vi "Auto State Machine.vi"   [LabVIEW 2013]
uses:
  typedefs/singleUseSubstate.ctl
  typedefs/subStates.ctl
  typedefs/DevRef Type.ctl
  typedefs/fg_typedef.ctl
  <vilib>/Rock Robotics/WPI/Solenoid/WPI_SolenoidValue.ctl
  <vilib>/Rock Robotics/WPI/Solenoid/WPI_SolenoidGetEnum.vi
panel:
  # "A State Machine to Handle One or Two Ball Autonomous"
types:
  T1 = typedef "singleUseSubstate.ctl" = enum16{"null", "wait", "shift high", "shift low", "extend shooter", "retract shooter", "latch", "unlatch"}
  T2 = typedef "subStates.ctl" = enum16{"null", "wait", "driver control", "auto", "manual override", "hold position", "rotate", "pickup", "pass", "load", "goto shoot", "shoot high goal", "shoot low goal", "cancel arm", "cancel shooter", "end"}
  T3 = typedef "WPI_SolenoidValue.ctl" = enum16{"Off", "On", "Forward", "Reverse"}
  T4 = typedef "DevRef Type.ctl" = enum16{"Shooter Solenoid", "Latch Solenoid", "Right Up Sensor", "Right Down Sensor", "Hold Sensor", "Arm Encoder"}
  T5 = typedef "fg_typedef.ctl" = enum16{"Get", "Set"}
  T6 = typedef "WPI_DigitalInputDevRef.ctl" = cluster{"DevStatus":errorcluster, "DIO Channel":T7, "Digital Module":T8}
  T7 = typedef "FPGA_DIOChannel.ctl" = enum8{"DIO 1", "DIO 2", "DIO 3", "DIO 4", "DIO 5", "DIO 6", "DIO 7", "DIO 8", "DIO 9", "DIO 10", "DIO 11", "DIO 12", "DIO 13", "DIO 14", "Invalid"}
  T8 = typedef "FPGA_TypedefDigitalModule.ctl" = enum16{"Digital Module 1", "Digital Module 2"}
  T9 = typedef "WPI_SolenoidDevRef.ctl" = cluster{"DevStatus":errorcluster, "Solenoid Module":T10, "Forward Solenoid Channel":T11, "Reverse Solenoid Channel":T11}
  T10 = typedef "FPGA_TypedefSolenoidModule.ctl" = enum16{"Solenoid Module 1", "Solenoid Module 2"}
  T11 = typedef "WPI_SolenoidChannel.ctl" = enum8{"Solenoid 1", "Solenoid 2", "Solenoid 3", "Solenoid 4", "Solenoid 5", "Solenoid 6", "Solenoid 7", "Solenoid 8", "Invalid"}
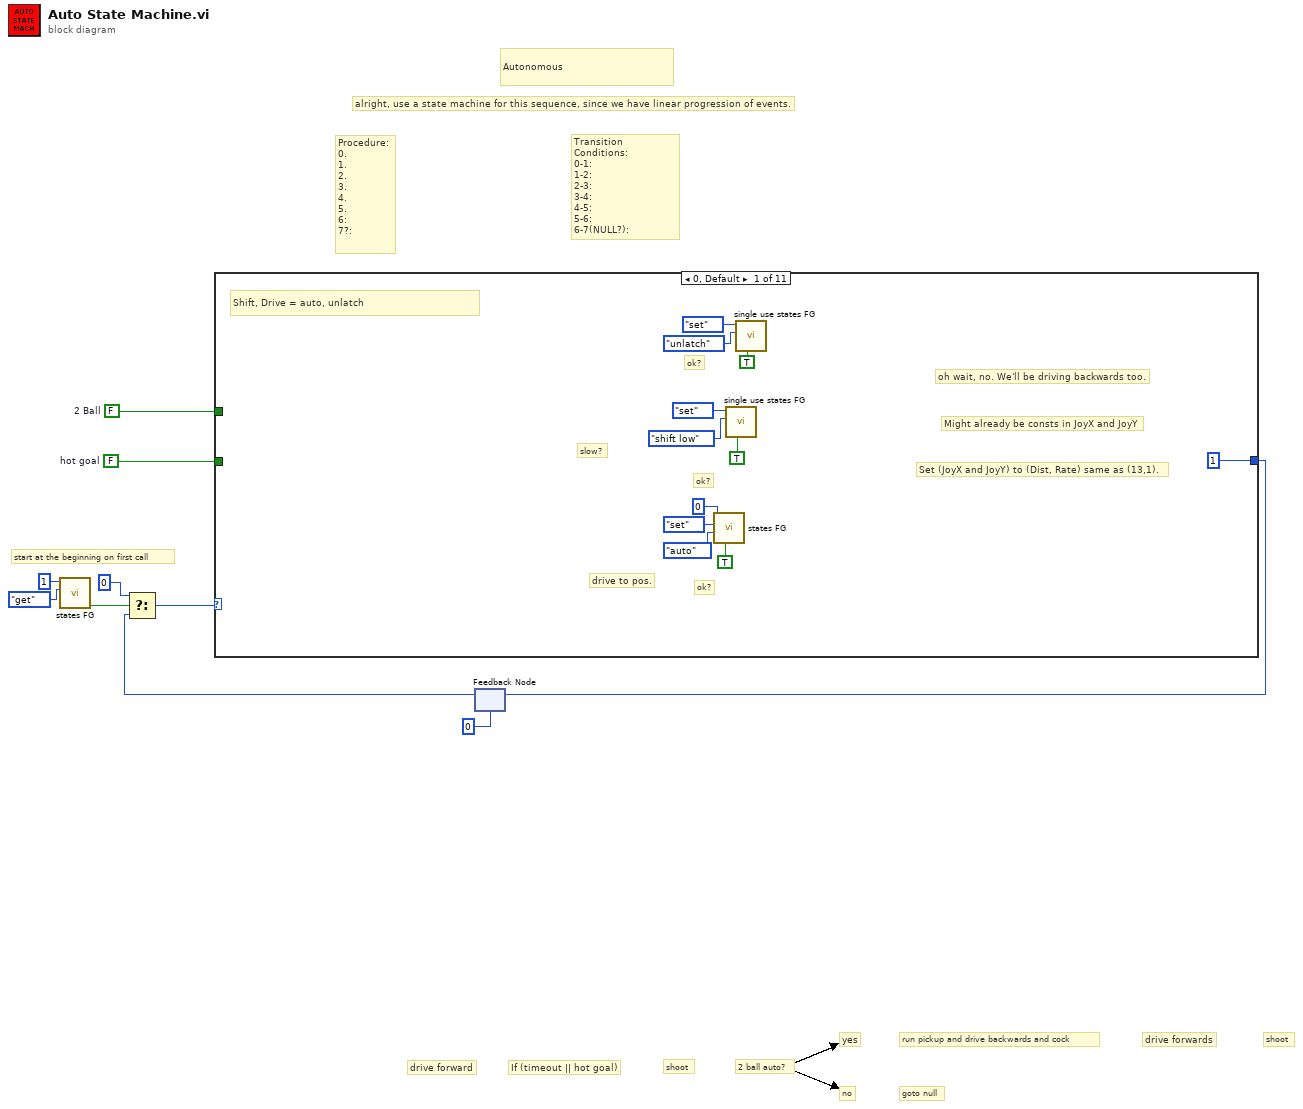
[diagram p0: block diagram]
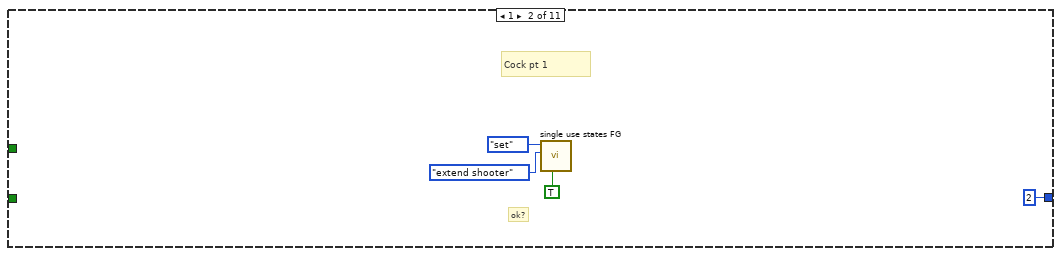
[diagram p2: hidden frame]
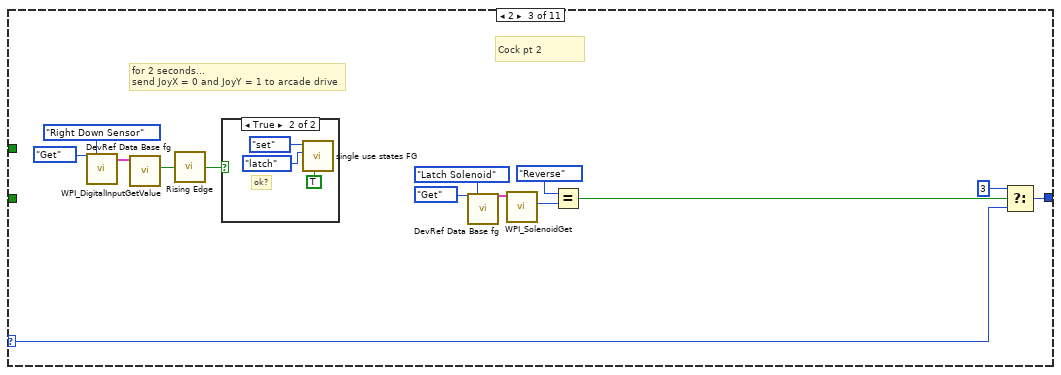
[diagram p3: hidden frame]
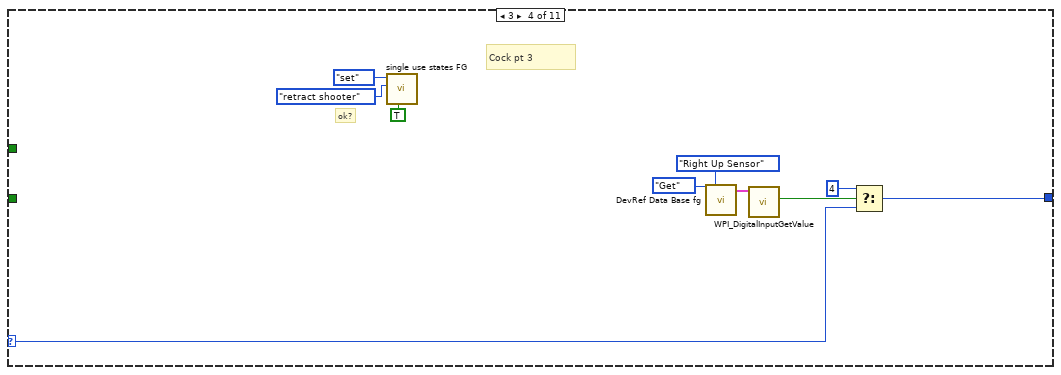
[diagram p5: hidden frame]
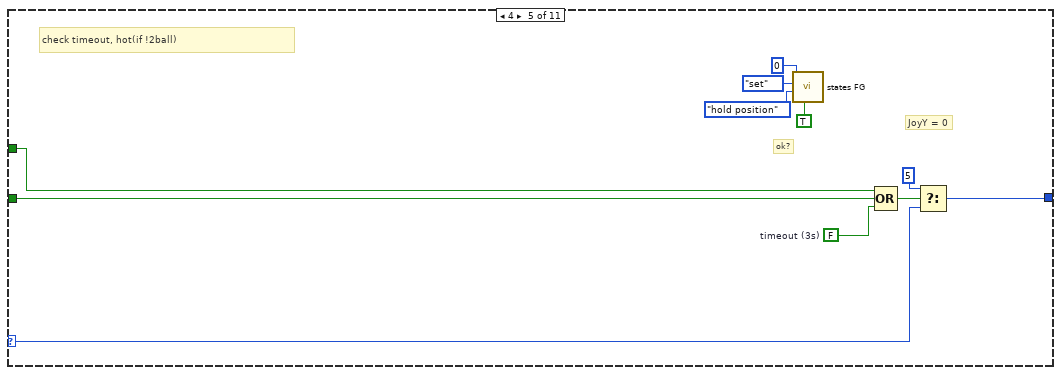
[diagram p6: hidden frame]
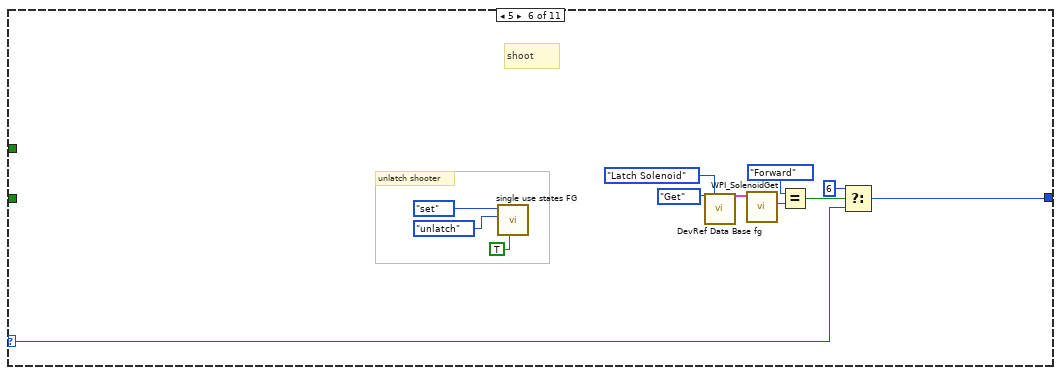
[diagram p7: hidden frame]
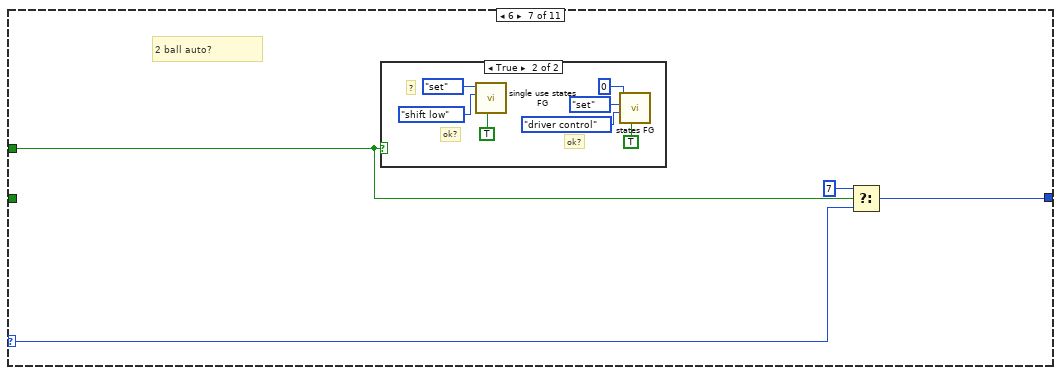
[diagram p8: hidden frame]
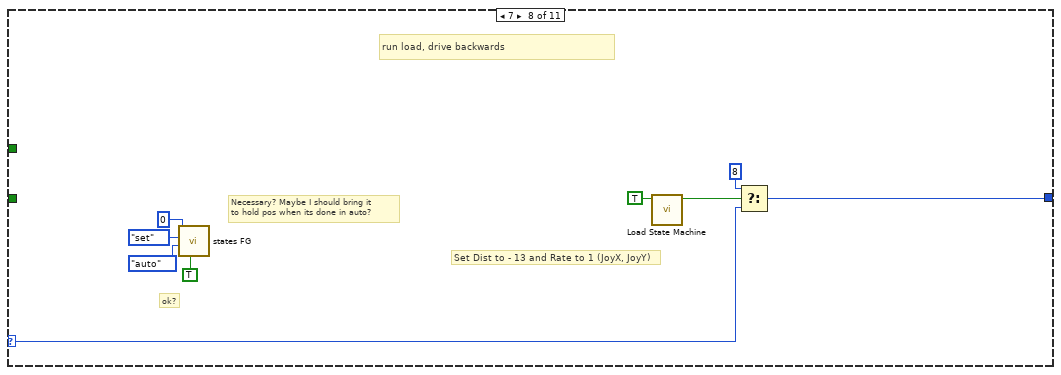
[diagram p10: hidden frame]
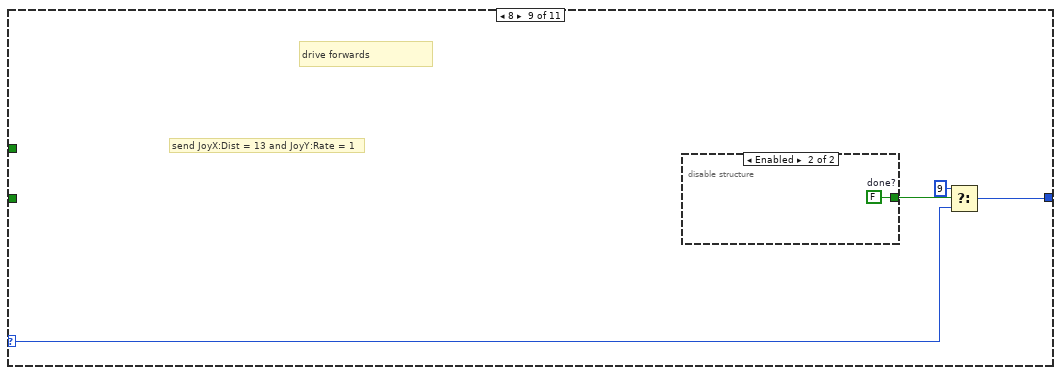
[diagram p11: hidden frame]
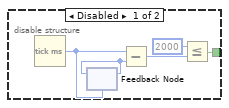
[diagram p12: hidden frame]
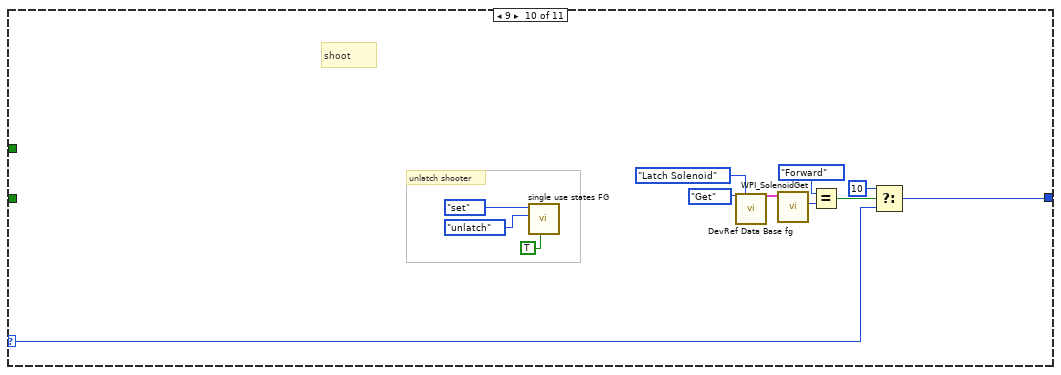
[diagram p13: hidden frame]
diagram:
  w3 = FALSE  # hot goal
  w4 = FALSE  # 2 Ball
  # "2 ball auto?"
  # "goto null"
  # "shoot"
  # "drive forwards"
  # "run pickup and drive backwards and cock"
  # "If (timeout || hot goal)"
  # "shoot"
  # "drive forward"
  # "no"
  # "yes"
  # "Transition Conditions:\n0-1: \n1-2: \n2-3: \n3-4: \n4-5: \n5-6:\n6-7(NULL?):"
  # "start at the beginning on first call"
  # "Autonomous"
  # "Procedure: \n0. \n1.\n2. \n3. \n4. \n5.\n6:\n7?:"
  # "alright, use a state machine for this sequence, since we have linear progression of events."
  n1 = call "states FG.vi"("menu (get)"=enum16{"set", "get"}."get", "Loop ID"=1) -> ("first call?"=w5:bool)  [unwired: 6 in, 3 out]
  n2 = feedback #1(u8 0) -> (w6:u8)
  n3 = Select(t=u8 0, s=w5, f=w6) -> (s? t:f=w8:u8)
  n4 = case shown="0, Default" w8 {
    selector: w8 -> [_ _ w39 w46 w63 w66 w79 w95 w97 w107 w118]
    tunnel: w4 -> [_ _ _ _ w59 _ w76 _ _ _ _]
    tunnel: w3 -> [_ _ _ _ w58 _ _ _ _ _ _]
    tunnel: [u8 1 u8 2 ("t") w38 w45 w57 w64 w77 w92 w96 w106 w118] -> w1
    frame 0, Default {
      # "oh wait, no. We'll be driving backwards too."
      # "Might already be consts in JoyX and JoyY"
      # "drive to pos."
      # "ok?"
      # "Shift, Drive = auto, unlatch"
      # "Set (JoyX and JoyY) to (Dist, Rate) same as (13,1)."
      # "ok?"
      # "ok?"
      # "slow?"
      n5 = call "states FG.vi"("exit in"=TRUE, "subState in"=subStates."auto", "menu (get)"=enum16{"set", "get"}."set", "Loop ID"=0) -> ()  [unwired: 4 in, 4 out]
      n6 = call "single use states FG.vi"("exit in"=TRUE, "substate"=singleUseSubstate."shift low", "menu (get)"=enum16{"set", "get"}."set") -> ()  [unwired: 5 in, 4 out]
      n7 = call "single use states FG.vi"("exit in"=TRUE, "substate"=singleUseSubstate."unlatch", "menu (get)"=enum16{"set", "get"}."set") -> ()  [unwired: 5 in, 4 out]
    }
    frame 1 {
      # "Cock pt 1"
      # "ok?"
      n8 = call "single use states FG.vi"("exit in"=TRUE, "substate"=singleUseSubstate."extend shooter", "menu (get)"=enum16{"set", "get"}."set") -> ()  [unwired: 5 in, 4 out]
    }
    frame 2 {
      # "for 2 seconds...\nsend JoyX = 0 and JoyY = 1 to arcade drive"
      # "Cock pt 2"
      n9 = call "DevRef Data Base fg.vi"("Menu"=fg_typedef."Get", "DevRef to Get"=DevRef_Type."Right Down Sensor") -> ("Selected Sensor"=w35:T6)  [unwired: 23 in, 2 out]
      n10 = call <vilib>:"WPI_DigitalInputGetValue.vi"("DigitalInputDevRef"=w35) -> ("Value"=w33:bool)  [unwired: 8 in, 2 out]
      n11 = call "Rising Edge.vi"("Input"=w33) -> ("Rising Edge"=w34:bool)
      n12 = case shown="True" w34 {
        frame False {
        }
        frame True {
          # "ok?"
          n13 = call "single use states FG.vi"("exit in"=TRUE, "substate"=singleUseSubstate."latch", "menu (get)"=enum16{"set", "get"}."set") -> ()  [unwired: 5 in, 4 out]
        }
      }
      n14 = call "DevRef Data Base fg.vi"("Menu"=fg_typedef."Get", "DevRef to Get"=DevRef_Type."Latch Solenoid") -> ("Selected Solenoid"=w30:T9)  [unwired: 23 in, 2 out]
      n15 = call-poly <vilib>:"WPI_SolenoidGet.vi"("SolenoidDevRef"=w30) -> ("Value"=w29:T3)  [unwired: 8 in, 2 out]
      n16 = Equal?(x=WPI_SolenoidValue."Reverse", y=w29) -> (x = y?=w26:bool)
      n17 = Select(t=u8 3, s=w26, f=w39) -> (s? t:f=w38:u8)
    }
    frame 3 {
      # "Cock pt 3"
      # "ok?"
      n18 = call "single use states FG.vi"("exit in"=TRUE, "substate"=singleUseSubstate."retract shooter", "menu (get)"=enum16{"set", "get"}."set") -> ()  [unwired: 5 in, 4 out]
      n19 = call "DevRef Data Base fg.vi"("Menu"=fg_typedef."Get", "DevRef to Get"=DevRef_Type."Right Up Sensor") -> ("Selected Sensor"=w47:T6)  [unwired: 23 in, 2 out]
      n20 = call <vilib>:"WPI_DigitalInputGetValue.vi"("DigitalInputDevRef"=w47) -> ("Value"=w44:bool)  [unwired: 8 in, 2 out]
      n21 = Select(t=u8 4, s=w44, f=w46) -> (s? t:f=w45:u8)
    }
    frame 4 {
      w60 = FALSE  # timeout (3s)
      # "ok?"
      # "JoyY = 0"
      # "check timeout, hot(if !2ball)"
      n22 = call "states FG.vi"("exit in"=TRUE, "subState in"=subStates."hold position", "menu (get)"=enum16{"set", "get"}."set", "Loop ID"=0) -> ()  [unwired: 4 in, 4 out]
      n23 = Compound Arithmetic op=OR(w59, w58, w60) -> (w61:bool)
      n24 = Select(t=u8 5, s=w61, f=w63) -> (s? t:f=w57:u8)
    }
    frame 5 {
      # "unlatch shooter"
      # "shoot"
      n25 = call "single use states FG.vi"("exit in"=TRUE, "substate"=singleUseSubstate."unlatch", "menu (get)"=enum16{"set", "get"}."set") -> ()  [unwired: 5 in, 4 out]
      n26 = call "DevRef Data Base fg.vi"("Menu"=fg_typedef."Get", "DevRef to Get"=DevRef_Type."Latch Solenoid") -> ("Selected Solenoid"=w71:T9)  [unwired: 23 in, 2 out]
      n27 = call-poly <vilib>:"WPI_SolenoidGet.vi"("SolenoidDevRef"=w71) -> ("Value"=w70:T3)  [unwired: 8 in, 2 out]
      n28 = Equal?(x=WPI_SolenoidValue."Forward" ("Value"), y=w70) -> (x = y?=w68:bool)
      n29 = Select(t=u8 6, s=w68, f=w66) -> (s? t:f=w64:u8)
    }
    frame 6 {
      # "2 ball auto?"
      n30 = case shown="True" w76 {
        frame False {
          # "goto null"
        }
        frame True {
          # "ok?"
          # "ok?"
          # "?"
          n31 = call "single use states FG.vi"("exit in"=TRUE, "substate"=singleUseSubstate."shift low", "menu (get)"=enum16{"set", "get"}."set") -> ()  [unwired: 5 in, 4 out]
          n32 = call "states FG.vi"("exit in"=TRUE, "subState in"=subStates."driver control", "menu (get)"=enum16{"set", "get"}."set", "Loop ID"=0) -> ()  [unwired: 4 in, 4 out]
        }
      }
      n33 = Select(t=u8 7, s=w76, f=w79) -> (s? t:f=w77:u8)
    }
    frame 7 {
      # "Set Dist to - 13 and Rate to 1 (JoyX, JoyY)"
      # "Necessary? Maybe I should bring it\nto hold pos when its done in auto?"
      # "ok?"
      # "run load, drive backwards"
      n34 = call "states FG.vi"("exit in"=TRUE, "subState in"=subStates."auto", "menu (get)"=enum16{"set", "get"}."set", "Loop ID"=0) -> ()  [unwired: 4 in, 4 out]
      n35 = call "Load State Machine.vi"("Autonomous? (Default false)"=TRUE ("Autonomous?")) -> ("Done (For Auto Use Only)"=w87:bool)  [unwired: 10 in]
      n36 = Select(t=u8 8, s=w87, f=w95) -> (s? t:f=w92:u8)
    }
    frame 8 {
      # "send JoyX:Dist = 13 and JoyY:Rate = 1"
      # "drive forwards"
      n37 = disable-structure shown="Enabled" {
        disable-tunnel: [w100 w105] -> w99
        frame Disabled {
          n38 = Tick Count (ms)() -> (millisecond timer value=w102:u32)
          n39 = feedback #2(w102) -> (w101:u32)
          n40 = feedback-in #2(w101) -> ()
          n41 = Subtract(x=w102, y=w101) -> (x-y=w104:u32)
          n42 = Less Or Equal?(x=u32 2000, y=w104) -> (x <= y?=w100:bool)
        }
        frame Enabled {
          w105 = FALSE  # done?
        }
      }
      n43 = Select(t=u8 9, s=w99, f=w97) -> (s? t:f=w96:u8)
    }
    frame 9 {
      # "unlatch shooter"
      # "shoot"
      n44 = call "single use states FG.vi"("exit in"=TRUE, "substate"=singleUseSubstate."unlatch", "menu (get)"=enum16{"set", "get"}."set") -> ()  [unwired: 5 in, 4 out]
      n45 = call "DevRef Data Base fg.vi"("Menu"=fg_typedef."Get", "DevRef to Get"=DevRef_Type."Latch Solenoid") -> ("Selected Solenoid"=w113:T9)  [unwired: 23 in, 2 out]
      n46 = call-poly <vilib>:"WPI_SolenoidGet.vi"("SolenoidDevRef"=w113) -> ("Value"=w112:T3)  [unwired: 8 in, 2 out]
      n47 = Equal?(x=WPI_SolenoidValue."Forward" ("Value"), y=w112) -> (x = y?=w110:bool)
      n48 = Select(t=u8 10, s=w110, f=w107) -> (s? t:f=w106:u8)
    }
    frame 10 {
      # "goto null?"
    }
  }
  n49 = feedback-in #1(w1) -> ()
